vi "getOpeningPercentage.vi"(8 "error in (no error)":errorcluster, 11 "DomeController in":refnum<class "DomeController.lvclass">) -> (0 "error out":errorcluster, 2 "openingPercentage":T1 min=0.0 max=100.0, 3 "DomeController out":refnum<class "DomeController.lvclass">)   [LabVIEW 2016, in "DomeController.lvclass"]
uses:
  DomeController.lvclass
  IDome/domeTypedefs/openingPercentage.ctl
  DomeController.lvclass/DomeController.ctl
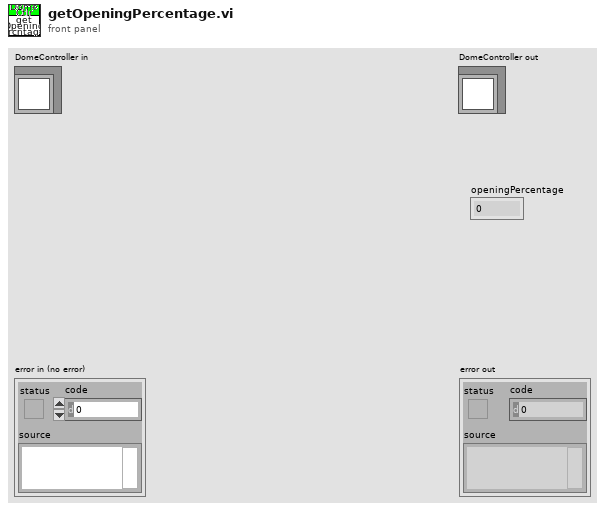
[diagram p1: front panel]
types:
  T1 = typedef "openingPercentage.ctl" = dbl
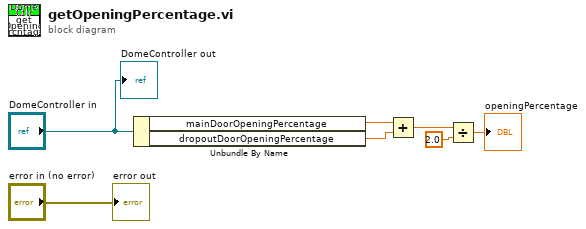
[diagram p0: block diagram]
diagram:
  n1 = Unbundle By Name("DomeController in") -> ("mainDoorOpeningPercentage"=w5:T1, "dropoutDoorOpeningPercentage"=w4:T1)
  n2 = Add(x=w5, y=w4) -> (x+y=w3:T1)
  n3 = Divide(x=w3, y=T1 2.0) -> (x/y=→"openingPercentage":T1)
  "error out" <- "error in (no error)"
  "DomeController out" <- "DomeController in"
